vi "daq_multi_output.vi"() -> ()   [LabVIEW 2017]
uses:
  <vilib>/Utility/file.llb/Read Delimited Spreadsheet (DBL).vi
  <vilib>/Analysis/NI_AALBase.lvlib
panel:
  in  "Reduce Amplitude":bool
  out "Waveform Graph":waveform(dbl)(graph)
  out "Length of Channel 4":dbl
  out "Length of Channel 2":dbl
  out "Length of Channel 6":dbl
  out "Length of Channel 5":dbl
  out "Length of Channel 1":dbl
  out "Length of Channel 7":dbl
  out "Matrix Cols 2":dbl
  out "Matrix Rows 2":dbl
  out "Length of Channel 0":dbl
  out "Length of Square Wave":dbl
  out "Data Max Val":dbl
  out "Matrix Cols":dbl
  out "Matrix Rows":dbl
  in  "stop (F)":bool
  in  "csv Path":path
  # "This .vi is for a single data waveform .wav output to 8 analog output channels"
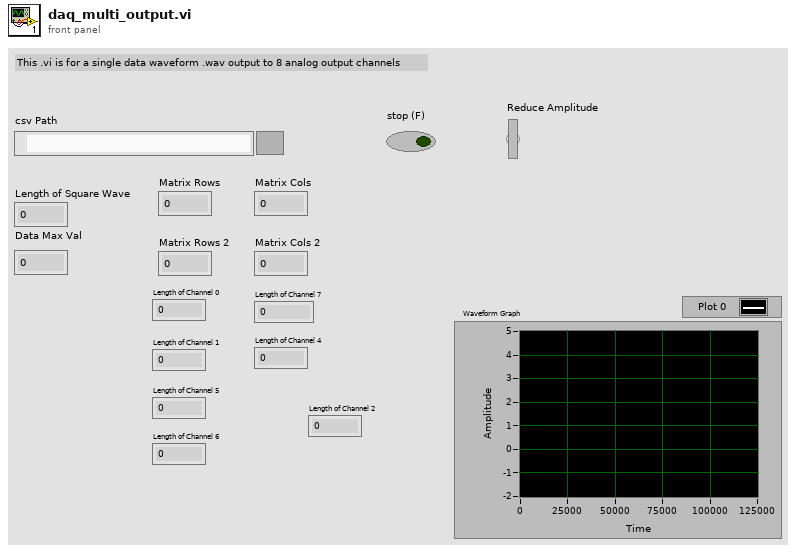
[diagram p1: front panel]
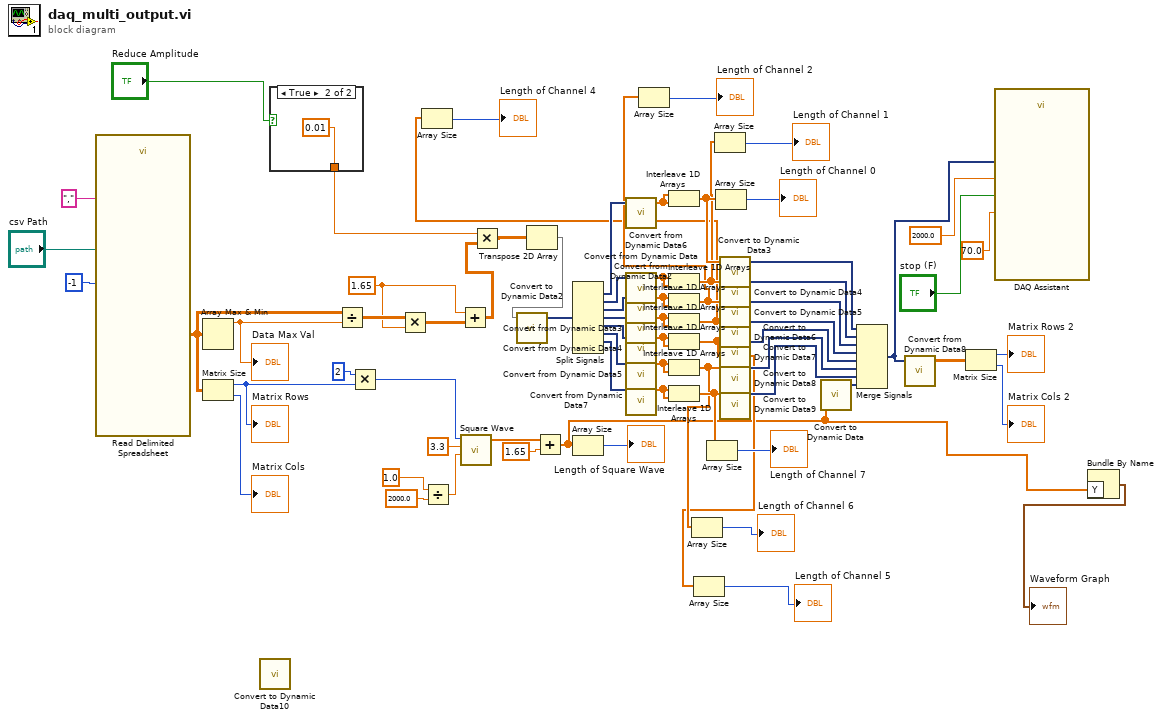
[diagram p0: block diagram]
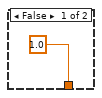
[diagram p2: hidden frame]
diagram:
  w59 = 1.65
  n1 = call-poly <vilib>:"Read Delimited Spreadsheet.vi"("file path (dialog if empty)"="csv Path", "number of rows (all:-1)"=-1, "delimiter (\\t)"=",") -> ("all rows"=w62:dbl[][])  [unwired: 7 in, 5 out]
  n2 = Array Max & Min(array=w62) -> (max value=w61:dbl)  [unwired: 3 out]
  "Data Max Val" <- w61
  n3 = Matrix Size(0:w62) -> (1:w26:i32, 2:→"Matrix Cols":i32)
  "Matrix Rows" <- w26
  n4 = call "Convert to Dynamic Data10"() -> ()  [unwired: 4 in, 1 out]
  n5 = case shown="True" "Reduce Amplitude" {
    tunnel: [1.0 0.01] -> w1
    frame False {
    }
    frame True {
    }
  }
  n6 = Divide(x=w62, y=w61) -> (x/y=w66:dbl[][])
  n7 = Multiply(x=2, y=w26) -> (x*y=w25:i32)
  n8 = Multiply(x=w66, y=w59) -> (x*y=w60:dbl[][])
  n9 = Divide(x=1.0, y=2000.0) -> (x/y=w31:dbl)
  n10 = Add(x=w59, y=w60) -> (x+y=w4:dbl[][])
  n11 = call <vilib>:"Square Wave.vi"("samples"=w25, "amplitude"=3.3, "frequency"=w31) -> ("square wave"=w34:dbl[])  [unwired: 3 in, 2 out]
  n12 = Multiply(x=w1, y=w4) -> (x*y=w3:dbl[][])
  n13 = Transpose 2D Array(2D array=w3) -> (transposed array=w21:dbl[][])
  n14 = call "Convert to Dynamic Data2"("2D Array"=w21) -> ("Dynamic Data Type"=w58:dynamicdata)  [unwired: 3 in]
  n15 = Add(x=w34, y=1.65) -> (x+y=w6:dbl[])
  n16 = Split Signals(w58) -> (w50:dynamicdata, w57:dynamicdata, w49:dynamicdata, w48:dynamicdata, w47:dynamicdata, w46:dynamicdata, w44:dynamicdata)  [unwired: 9 in, 2 out]
  n17 = Array Size(array=w6) -> (size(s)=→"Length of Square Wave":i32)
  n18 = call "Convert from Dynamic Data6"("Dynamic Data Type"=w50) -> ("Array"=w51:dbl[])  [unwired: 3 in]
  n19 = call "Convert from Dynamic Data"("Dynamic Data Type"=w57) -> ("Array"=w56:dbl[])  [unwired: 3 in]
  n20 = call "Convert from Dynamic Data2"("Dynamic Data Type"=w49) -> ("Array"=w55:dbl[])  [unwired: 3 in]
  n21 = call "Convert from Dynamic Data3"("Dynamic Data Type"=w48) -> ("Array"=w54:dbl[])  [unwired: 3 in]
  n22 = call "Convert from Dynamic Data4"("Dynamic Data Type"=w47) -> ("Array"=w53:dbl[])  [unwired: 3 in]
  n23 = call "Convert from Dynamic Data5"("Dynamic Data Type"=w46) -> ("Array"=w52:dbl[])  [unwired: 3 in]
  n24 = call "Convert from Dynamic Data7"("Dynamic Data Type"=w44) -> ("Array"=w45:dbl[])  [unwired: 3 in]
  n25 = Interleave 1D Arrays(w51, w51) -> (w28:dbl[])
  n26 = Interleave 1D Arrays(w56, w56) -> (w17:dbl[])
  n27 = Interleave 1D Arrays(w55, w55) -> (w11:dbl[])
  n28 = Array Size(array=w11) -> (size(s)=→"Length of Channel 2":i32)
  n29 = Interleave 1D Arrays(w54, w54) -> (w8:dbl[])
  n30 = Array Size(array=w8) -> (size(s)=→"Length of Channel 4":i32)
  n31 = Interleave 1D Arrays(w53, w53) -> (w13:dbl[])
  n32 = Interleave 1D Arrays(w52, w52) -> (w15:dbl[])
  n33 = Interleave 1D Arrays(w45, w45) -> (w19:dbl[])
  n34 = Array Size(array=w15) -> (size(s)=→"Length of Channel 6":i32)
  n35 = Array Size(array=w13) -> (size(s)=→"Length of Channel 5":i32)
  n36 = Array Size(array=w19) -> (size(s)=→"Length of Channel 7":i32)
  n37 = Array Size(array=w17) -> (size(s)=→"Length of Channel 1":i32)
  n38 = Array Size(array=w28) -> (size(s)=→"Length of Channel 0":i32)
  n39 = call "Convert to Dynamic Data3"("Array"=w28) -> ("Dynamic Data Type"=w43:dynamicdata)  [unwired: 3 in]
  n40 = call "Convert to Dynamic Data4"("Array"=w17) -> ("Dynamic Data Type"=w42:dynamicdata)  [unwired: 3 in]
  n41 = call "Convert to Dynamic Data5"("Array"=w11) -> ("Dynamic Data Type"=w41:dynamicdata)  [unwired: 3 in]
  n42 = call "Convert to Dynamic Data6"("Array"=w8) -> ("Dynamic Data Type"=w40:dynamicdata)  [unwired: 3 in]
  n43 = call "Convert to Dynamic Data7"("Array"=w13) -> ("Dynamic Data Type"=w39:dynamicdata)  [unwired: 3 in]
  n44 = call "Convert to Dynamic Data8"("Array"=w15) -> ("Dynamic Data Type"=w38:dynamicdata)  [unwired: 3 in]
  n45 = call "Convert to Dynamic Data9"("Array"=w19) -> ("Dynamic Data Type"=w37:dynamicdata)  [unwired: 3 in]
  n46 = call "Convert to Dynamic Data"("Array"=w6) -> ("Dynamic Data Type"=w9:dynamicdata)  [unwired: 3 in]
  n47 = Merge Signals(w43, w42, w41, w40, w39, w38, w37, w9) -> (w24:dynamicdata)
  n48 = call "Convert from Dynamic Data8"("Dynamic Data Type"=w24) -> ("Array"=w5:dbl[][])  [unwired: 3 in]
  n49 = Matrix Size(0:w5) -> (1:→"Matrix Rows 2":i32, 2:→"Matrix Cols 2":i32)
  n50 = call "DAQ Assistant"("data"=w24, "rate"=2000.0, "timeout (s)"=70.0, "stop (T)"="stop (F)") -> ()  [unwired: 14 in, 2 out]
  n51 = Bundle By Name("Y"=w6) -> (→"Waveform Graph":waveform(dbl))  [unwired: 1 in]
